vi "Get square info.vi"(10 "Square":T1={"File"=enum."a", "Rank"=enum."4"}, 11 "Board in":refnum<class "Board.lvclass">) -> (1 "Piece":refnum<class "Piece.lvclass">, 2 "Square occupied?":bool, 3 "Board out":refnum<class "Board.lvclass">)   [LabVIEW 2016, in "Chesslib.lvlib" / "Board.lvclass"]
uses:
  Board.lvclass
  typedef/Square.ctl
  typedef/File.ctl
  typedef/Rank.ctl
  Pieces/Piece/Piece.lvclass
  Board.lvclass/Board.ctl
  Chesslib.lvlib
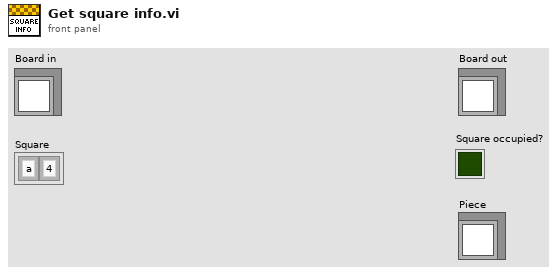
[diagram p1: front panel]
types:
  T1 = typedef "Chesslib.lvlib/Square.ctl" = cluster{"File":T2, "Rank":T3}
  T2 = typedef "Chesslib.lvlib/File.ctl" = enum8{"a", "b", "c", "d", "e", "f", "g", "h"}
  T3 = typedef "Chesslib.lvlib/Rank.ctl" = enum8{"1", "2", "3", "4", "5", "6", "7", "8"}
  T4 = typedef "Chesslib.lvlib/Board.lvclass/Square content.ctl" = cluster{"Occupied":bool, "Piece":refnum<class "Piece.lvclass">}
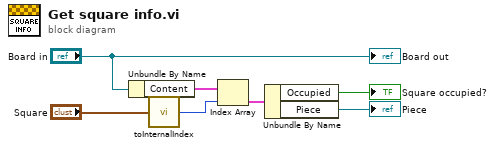
[diagram p0: block diagram]
diagram:
  n1 = Unbundle By Name("Board in") -> ("Content"=w5:T4[])
  n2 = call "toInternalIndex.vi"("Square"="Square") -> ("Internal index"=w6:u8)
  n3 = Index Array(array=w5, index=w6) -> (element=w3:T4)
  n4 = Unbundle By Name(w3) -> ("Occupied"=→"Square occupied?":bool, "Piece"=→"Piece":refnum<class "Piece.lvclass">)
  "Board out" <- "Board in"
